vi "Kalkulator.vi"() -> ()   [LabVIEW 2021]
uses:
  sm_data.ctl
panel:
  in  "Inwersja":bool
  in  "Kwadrat":bool
  in  "Negacja":bool
  in  "Pierwiastek":bool
  in  "C":bool
  in  "Enter":bool
  in  "X":dbl
  out "Z":dbl
  out "Y":dbl
  in  "Coma":bool
  in  "Dzielenie":bool
  in  "Mnożenie":bool
  in  "Odejmowanie":bool
  in  "Dodawanie":bool
  in  "0":bool
  in  "9":bool
  in  "8":bool
  in  "7":bool
  in  "6":bool
  in  "5":bool
  in  "4":bool
  in  "3":bool
  in  "2":bool
  in  "1":bool
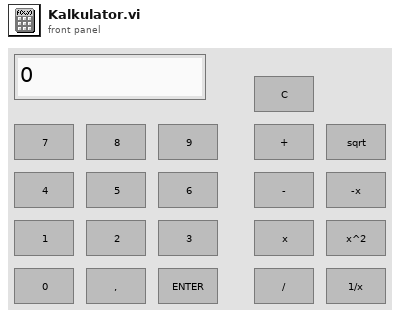
[diagram p1: front panel]
types:
  T1 = typedef "sm_data.ctl" = cluster{"number_str":string}
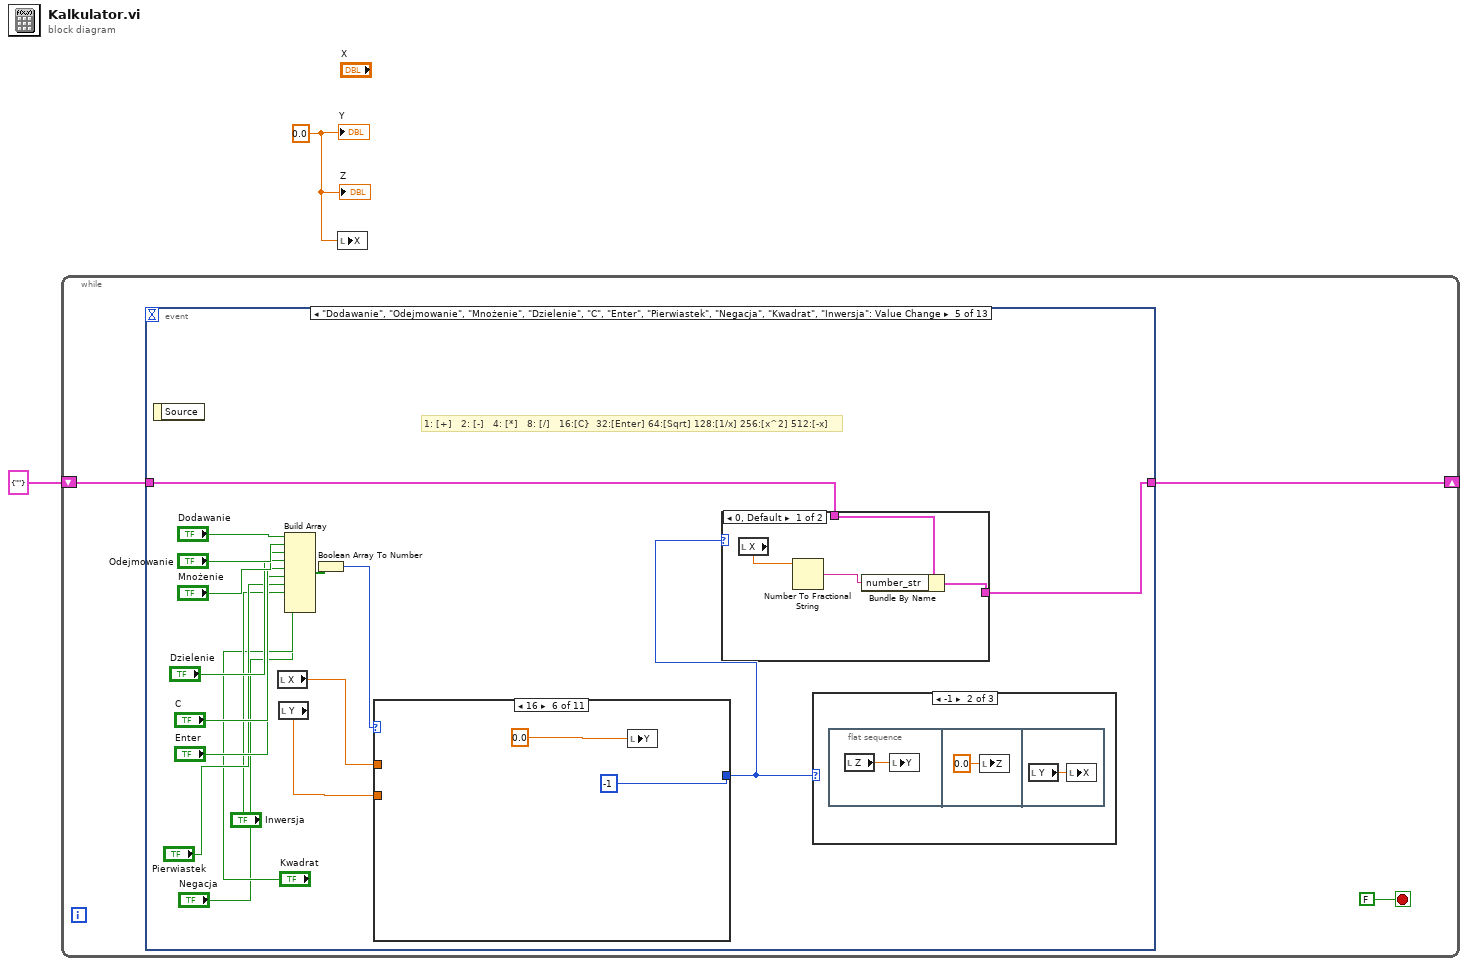
[diagram p0: block diagram]
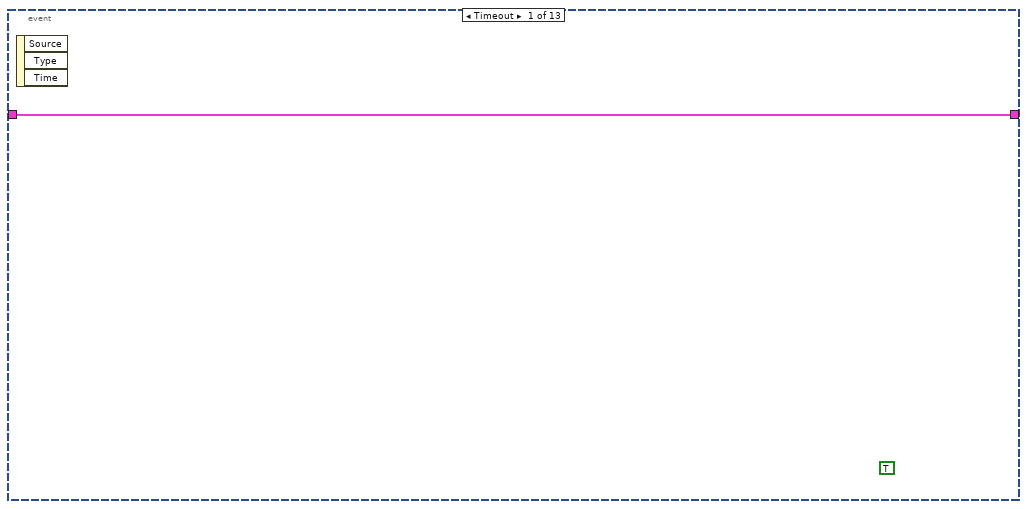
[diagram p2: hidden frame]
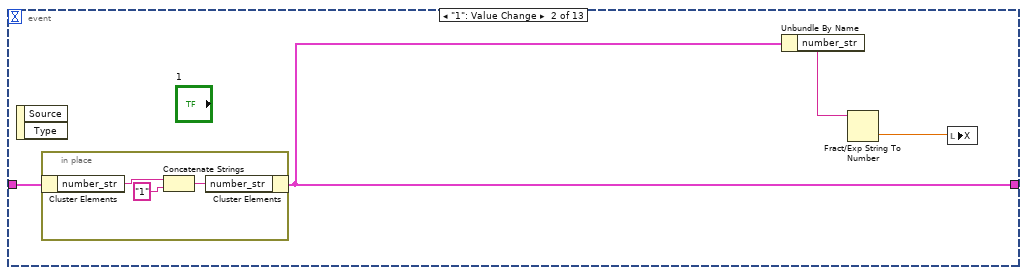
[diagram p3: hidden frame]
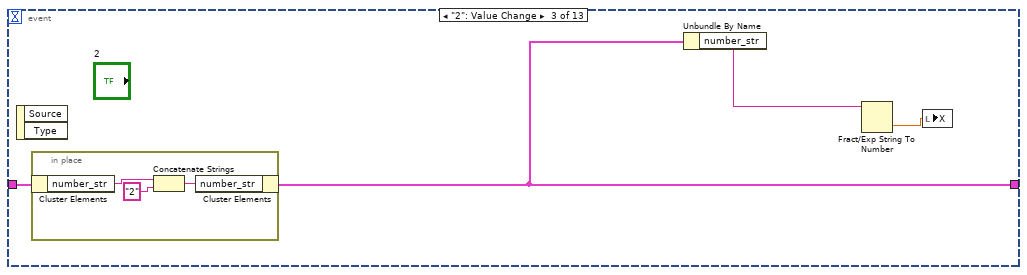
[diagram p4: hidden frame]
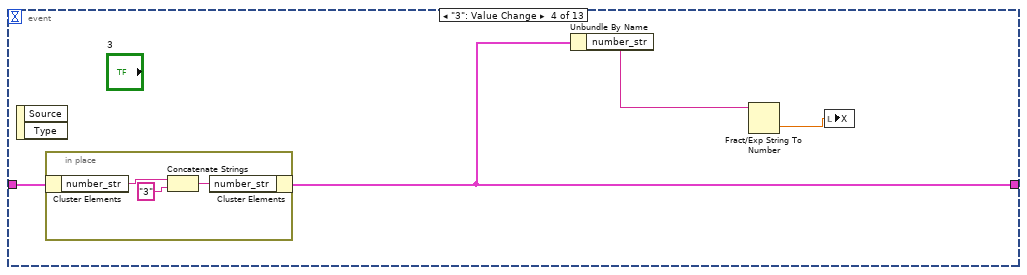
[diagram p5: hidden frame]
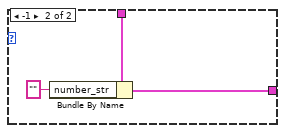
[diagram p6: hidden frame]
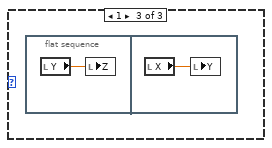
[diagram p8: hidden frame]
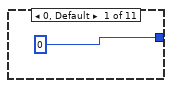
[diagram p9: hidden frame]
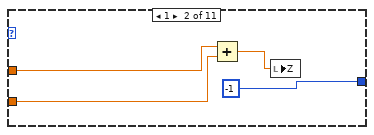
[diagram p10: hidden frame]
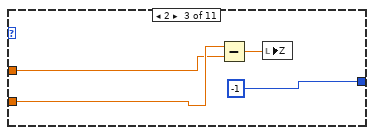
[diagram p11: hidden frame]
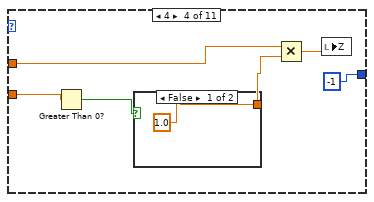
[diagram p12: hidden frame]
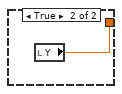
[diagram p13: hidden frame]
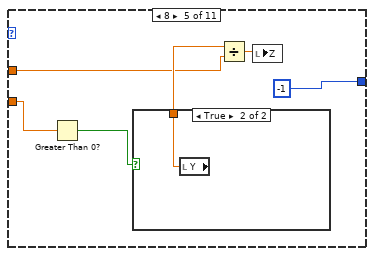
[diagram p14: hidden frame]
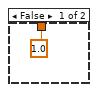
[diagram p15: hidden frame]
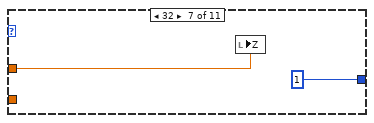
[diagram p16: hidden frame]
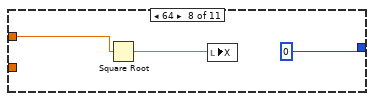
[diagram p17: hidden frame]
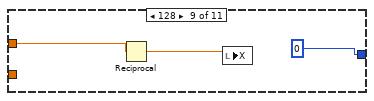
[diagram p18: hidden frame]
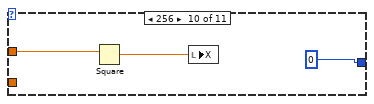
[diagram p19: hidden frame]
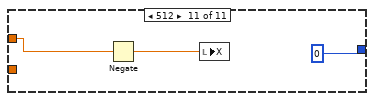
[diagram p20: hidden frame]
diagram:
  w1 = 0.0 ("Y")
  n1 = while {
    shift-right: [w4] -> _
    shift-left: T1 {"number_str"=""} -> [w5]
    stop <- FALSE stop-if-true
    n2 = event shown="[4] \"Dodawanie\", \"Odejmowanie\", \"Mnożenie\", \"Dzielenie\", \"C\", \"Enter\", \"Pierwiastek\", \"Negacja\", \"Kwadrat\", \"Inwersja\": Value Change" {
      selector: _ -> [_ _ _ _ _ _ _ _ _ _ _ _ _]
      dyn-events: _ -> [_ _ _ _ _ _ _ _ _ _ _ _ _]
      timeout: _ -> [_ _ _ _ _ _ _ _ _ _ _ _ _]
      tunnel: w5 -> [w6 w10 w17 w24 w30 w101 w108 w115 w122 w129 w136 w143 w150]
      tunnel: [w6 w9 w16 w22 w29 w99 w106 w113 w120 w127 w134 w141 w148] -> w4
      event Timeout {
        (unwired) TRUE
        n3 = event-data() -> ()  [unwired: 1 in, 3 out]
      }
      event "1": Value Change {
        n4 = event-data() -> ()  [unwired: 1 in, 2 out]
        n5 = in-place {
          n6 = in-place-cluster #1(w10) -> ("number_str"=w13:string)
          n7 = Concatenate Strings(w13, "1" ("string")) -> (w12:string)
          n8 = in-place-cluster #1("number_str"=w12) -> (w9:T1)
        }
        n9 = Unbundle By Name(w9) -> ("number_str"=w7:string)
        n10 = Fract/Exp String To Number(string=w7) -> (number=w8:dbl)  [unwired: 3 in, 1 out]
        n11 = local write "X"(w8) -> ()
      }
      event "2": Value Change {
        n12 = event-data() -> ()  [unwired: 1 in, 2 out]
        n13 = in-place {
          n14 = in-place-cluster #2(w17) -> ("number_str"=w20:string)
          n15 = Concatenate Strings(w20, "2" ("string")) -> (w19:string)
          n16 = in-place-cluster #2("number_str"=w19) -> (w16:T1)
        }
        n17 = Unbundle By Name(w16) -> ("number_str"=w15:string)
        n18 = Fract/Exp String To Number(string=w15) -> (number=w14:dbl)  [unwired: 3 in, 1 out]
        n19 = local write "X"(w14) -> ()
      }
      event "3": Value Change {
        n20 = event-data() -> ()  [unwired: 1 in, 2 out]
        n21 = in-place {
          n22 = in-place-cluster #3(w24) -> ("number_str"=w27:string)
          n23 = Concatenate Strings(w27, "3" ("string")) -> (w26:string)
          n24 = in-place-cluster #3("number_str"=w26) -> (w22:T1)
        }
        n25 = Unbundle By Name(w22) -> ("number_str"=w23:string)
        n26 = Fract/Exp String To Number(string=w23) -> (number=w21:dbl)  [unwired: 3 in, 1 out]
        n27 = local write "X"(w21) -> ()
      }
      event "Dodawanie", "Odejmowanie", "Mnożenie", "Dzielenie", "C", "Enter", "Pierwiastek", "Negacja", "Kwadrat", "Inwersja": Value Change {
        # "1: [+]   2: [-]   4: [*]   8: [/]   16:[C}  32:[Enter] 64:[Sqrt] 128:[1/x] 256:[x^2] 512:[-x]"
        n28 = event-data() -> ()  [unwired: 1 in, 1 out]
        n29 = local read "X"() -> (w38:dbl)
        n30 = local read "Y"() -> (w39:dbl)
        n31 = Build Array("Dodawanie", "Odejmowanie", "Mnożenie", "Dzielenie", "C", "Enter", "Pierwiastek", "Inwersja", "Kwadrat", "Negacja") -> (w44:bool[])
        n32 = Boolean Array To Number(Boolean array=w44) -> (number=w37:u32)
        n33 = case shown="16" w37 {
          tunnel: w39 -> [_ w61 w65 w67 w77 _ _ _ _ _ _]
          tunnel: w38 -> [_ w60 w64 w71 w74 _ w84 w87 w90 w93 w96]
          tunnel: [0 -1 -1 -1 -1 -1 1 0 0 0 0] -> w28
          frame 0, Default {
          }
          frame 1 {
            n34 = Add(x=w60, y=w61) -> (x+y=w58:dbl)
            n35 = local write "Z"(w58) -> ()
          }
          frame 2 {
            n36 = Subtract(x=w65, y=w64) -> (x-y=w62:dbl)
            n37 = local write "Z"(w62) -> ()
          }
          frame 4 {
            n38 = Greater Than 0?(x=w67) -> (x > 0?=w66:bool)
            n39 = case shown="False" w66 {
              tunnel: [1.0 ("y") w73] -> w68
              frame False {
              }
              frame True {
                n40 = local read "Y"() -> (w73:dbl)
              }
            }
            n41 = Multiply(x=w71, y=w68) -> (x*y=w69:dbl)
            n42 = local write "Z"(w69) -> ()
          }
          frame 8 {
            n43 = Greater Than 0?(x=w77) -> (x > 0?=w76:bool)
            n44 = case shown="True" w76 {
              tunnel: [1.0 ("Y") w81] -> w75
              frame False {
              }
              frame True {
                n45 = local read "Y"() -> (w81:dbl)
              }
            }
            n46 = Divide(x=w75, y=w74) -> (x/y=w78:dbl)
            n47 = local write "Z"(w78) -> ()
          }
          frame 16 {
            n48 = local write "Y"(0.0 ("Y")) -> ()
          }
          frame 32 {
            n49 = local write "Z"(w84) -> ()
          }
          frame 64 {
            n50 = Square Root(x=w87) -> (sqrt(x)=w86:dbl)
            n51 = local write "X"(w86) -> ()
          }
          frame 128 {
            n52 = Reciprocal(x=w90) -> (1/x=w89:dbl)
            n53 = local write "X"(w89) -> ()
          }
          frame 256 {
            n54 = Square(x=w93) -> (x^2=w92:dbl)
            n55 = local write "X"(w92) -> ()
          }
          frame 512 {
            n56 = Negate(x=w96) -> (-x=w95:dbl)
            n57 = local write "X"(w95) -> ()
          }
        }
        n58 = case shown="0, Default" w28 {
          tunnel: w30 -> [w46 w51]
          tunnel: [w47 w49] -> w29
          frame 0, Default {
            n59 = local read "X"() -> (w48:dbl)
            n60 = Number To Fractional String(number=w48) -> (F-format string=w45:string)  [unwired: 3 in]
            n61 = Bundle By Name(cluster=w46, "number_str"=w45) -> (w47:T1)
          }
          frame -1 {
            n62 = Bundle By Name(cluster=w51, "number_str"="") -> (w49:T1)
          }
        }
        n63 = case shown="-1" w28 {
          frame 0, Default {
          }
          frame -1 {
            n64 = flat-sequence {
              frame #0 {
                n65 = local read "Z"() -> (w52:dbl)
                n66 = local write "Y"(w52) -> ()
              }
              frame #1 {
                n67 = local write "Z"(0.0 ("Y")) -> ()
              }
              frame #2 {
                n68 = local read "Y"() -> (w54:dbl)
                n69 = local write "X"(w54) -> ()
              }
            }
          }
          frame 1 {
            n70 = flat-sequence {
              frame #0 {
                n71 = local read "Y"() -> (w55:dbl)
                n72 = local write "Z"(w55) -> ()
              }
              frame #1 {
                n73 = local read "X"() -> (w56:dbl)
                n74 = local write "Y"(w56) -> ()
              }
            }
          }
        }
      }
      event "4": Value Change {
        n75 = event-data() -> ()  [unwired: 1 in, 2 out]
        n76 = in-place {
          n77 = in-place-cluster #4(w101) -> ("number_str"=w104:string)
          n78 = Concatenate Strings(w104, "4" ("string")) -> (w103:string)
          n79 = in-place-cluster #4("number_str"=w103) -> (w99:T1)
        }
        n80 = Unbundle By Name(w99) -> ("number_str"=w100:string)
        n81 = Fract/Exp String To Number(string=w100) -> (number=w98:dbl)  [unwired: 3 in, 1 out]
        n82 = local write "X"(w98) -> ()
      }
      event "5": Value Change {
        n83 = event-data() -> ()  [unwired: 1 in, 2 out]
        n84 = in-place {
          n85 = in-place-cluster #5(w108) -> ("number_str"=w111:string)
          n86 = Concatenate Strings(w111, "5" ("string")) -> (w110:string)
          n87 = in-place-cluster #5("number_str"=w110) -> (w106:T1)
        }
        n88 = Unbundle By Name(w106) -> ("number_str"=w107:string)
        n89 = Fract/Exp String To Number(string=w107) -> (number=w105:dbl)  [unwired: 3 in, 1 out]
        n90 = local write "X"(w105) -> ()
      }
      event "6": Value Change {
        n91 = event-data() -> ()  [unwired: 1 in, 1 out]
        n92 = in-place {
          n93 = in-place-cluster #6(w115) -> ("number_str"=w118:string)
          n94 = Concatenate Strings(w118, "6" ("string")) -> (w117:string)
          n95 = in-place-cluster #6("number_str"=w117) -> (w113:T1)
        }
        n96 = Unbundle By Name(w113) -> ("number_str"=w114:string)
        n97 = Fract/Exp String To Number(string=w114) -> (number=w112:dbl)  [unwired: 3 in, 1 out]
        n98 = local write "X"(w112) -> ()
      }
      event "7": Value Change {
        n99 = event-data() -> ()  [unwired: 1 in, 2 out]
        n100 = in-place {
          n101 = in-place-cluster #7(w122) -> ("number_str"=w125:string)
          n102 = Concatenate Strings(w125, "7" ("string")) -> (w124:string)
          n103 = in-place-cluster #7("number_str"=w124) -> (w120:T1)
        }
        n104 = Unbundle By Name(w120) -> ("number_str"=w121:string)
        n105 = Fract/Exp String To Number(string=w121) -> (number=w119:dbl)  [unwired: 3 in, 1 out]
        n106 = local write "X"(w119) -> ()
      }
      event "8": Value Change {
        n107 = event-data() -> ()  [unwired: 1 in, 2 out]
        n108 = in-place {
          n109 = in-place-cluster #8(w129) -> ("number_str"=w132:string)
          n110 = Concatenate Strings(w132, "8" ("string")) -> (w131:string)
          n111 = in-place-cluster #8("number_str"=w131) -> (w127:T1)
        }
        n112 = Unbundle By Name(w127) -> ("number_str"=w128:string)
        n113 = Fract/Exp String To Number(string=w128) -> (number=w126:dbl)  [unwired: 3 in, 1 out]
        n114 = local write "X"(w126) -> ()
      }
      event "9": Value Change {
        n115 = event-data() -> ()  [unwired: 1 in, 1 out]
        n116 = in-place {
          n117 = in-place-cluster #9(w136) -> ("number_str"=w139:string)
          n118 = Concatenate Strings(w139, "9" ("string")) -> (w138:string)
          n119 = in-place-cluster #9("number_str"=w138) -> (w134:T1)
        }
        n120 = Unbundle By Name(w134) -> ("number_str"=w135:string)
        n121 = Fract/Exp String To Number(string=w135) -> (number=w133:dbl)  [unwired: 3 in, 1 out]
        n122 = local write "X"(w133) -> ()
      }
      event "0": Value Change {
        n123 = event-data() -> ()  [unwired: 1 in, 1 out]
        n124 = in-place {
          n125 = in-place-cluster #10(w143) -> ("number_str"=w146:string)
          n126 = Concatenate Strings(w146, "0" ("string")) -> (w145:string)
          n127 = in-place-cluster #10("number_str"=w145) -> (w141:T1)
        }
        n128 = Unbundle By Name(w141) -> ("number_str"=w142:string)
        n129 = Fract/Exp String To Number(string=w142) -> (number=w140:dbl)  [unwired: 3 in, 1 out]
        n130 = local write "X"(w140) -> ()
      }
      event "Coma": Value Change {
        n131 = event-data() -> ()  [unwired: 1 in, 1 out]
        n132 = in-place {
          n133 = in-place-cluster #11(w150) -> ("number_str"=w153:string)
          n134 = Concatenate Strings(w153, "," ("string")) -> (w152:string)
          n135 = in-place-cluster #11("number_str"=w152) -> (w148:T1)
        }
        n136 = Unbundle By Name(w148) -> ("number_str"=w149:string)
        n137 = Fract/Exp String To Number(string=w149) -> (number=w147:dbl)  [unwired: 3 in, 1 out]
        n138 = local write "X"(w147) -> ()
      }
    }
  }
  n139 = local write "X"(w1) -> ()
  "Y" <- w1
  "Z" <- w1
